vi "S2C_Shared_Proc_ErrorTrap.vi"(8 "Error In":errorcluster, 10 "Command":string, 11 "Q-Ref":refnum<queue>) -> (0 "Error Out":errorcluster)   [LabVIEW 2024]
doc: "Detects an error and calls the error case to process the error."
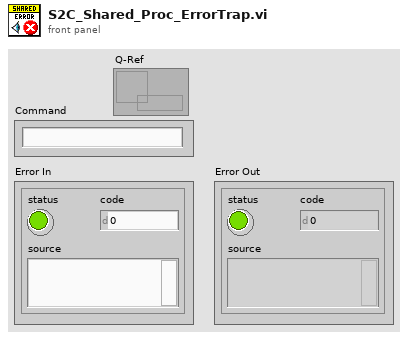
[diagram p1: front panel]
types:
  T1 = cluster{"Caller-Q":refnum<queue>, "Command":string, "Return":string, "Data":variant, "Timeout":dbl}
  T2 = cluster{"Command":string, "error IO":errorcluster}
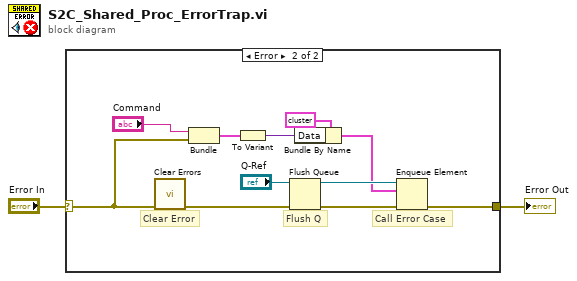
[diagram p0: block diagram]
diagram:
  n1 = case shown="Error" "Error In" {
    selector: "Error In" -> [w3 w6]
    tunnel: [w3 w11] -> w1
    frame No Error {
    }
    frame Error {
      # "Call Error Case"
      # "Flush Q"
      # "Clear Error"
      n2 = call <vilib>:"Clear Errors.vi"("error in (no error)"=w6) -> ("error out"=w14:errorcluster)  [unwired: 5 in, 1 out]
      n3 = Bundle("Command"="Command", "error IO"=w6) -> (w4:T2)  [unwired: 1 in]
      n4 = To Variant(anything=w4) -> (Variant=w8:variant)
      n5 = Flush Queue(queue="Q-Ref", error in (no error)=w14) -> (queue out=w12:refnum<queue>, error out=w13:errorcluster)  [unwired: 1 out]
      n6 = Bundle By Name(cluster=T1 {"Caller-Q"=refnum, "Command"="^Error", "Return"="None", "Data"=variant, "Timeout"=10.0} ("element"), "Data"=w8) -> (w7:T1)
      n7 = Enqueue Element(queue=w12, element=w7, error in (no error)=w13) -> (error out=w11:errorcluster)  [unwired: 1 in, 2 out]
    }
  }
  "Error Out" <- w1
